vi "GetNoOfFilesandIndices.vi"(8 "error in (no error)":errorcluster, 10 "Partial Image File Name":string="cameraA-nr", 11 "File Path":path=path "Z:/Downloads/Fridge Pictures/1") -> (0 "error out":errorcluster, 1 "Number of Files":i32, 2 "max value":i32, 3 "min value":i32, 4 "Index number of Files":i32[](array[numeric]), 5 "Dt":u32)   [LabVIEW 2013]
doc: "Use this template to build a VI to use as a subVI."
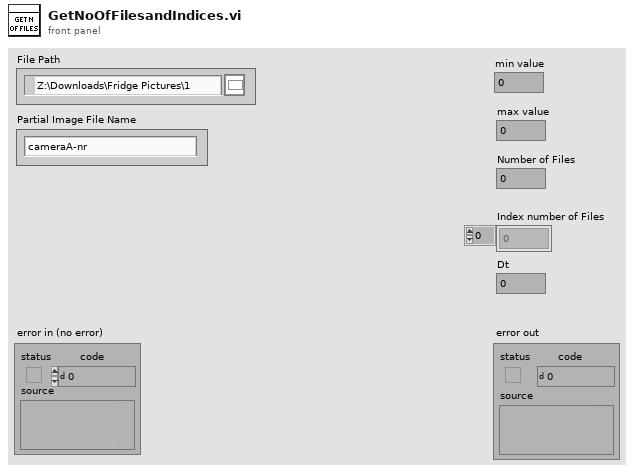
[diagram p1: front panel]
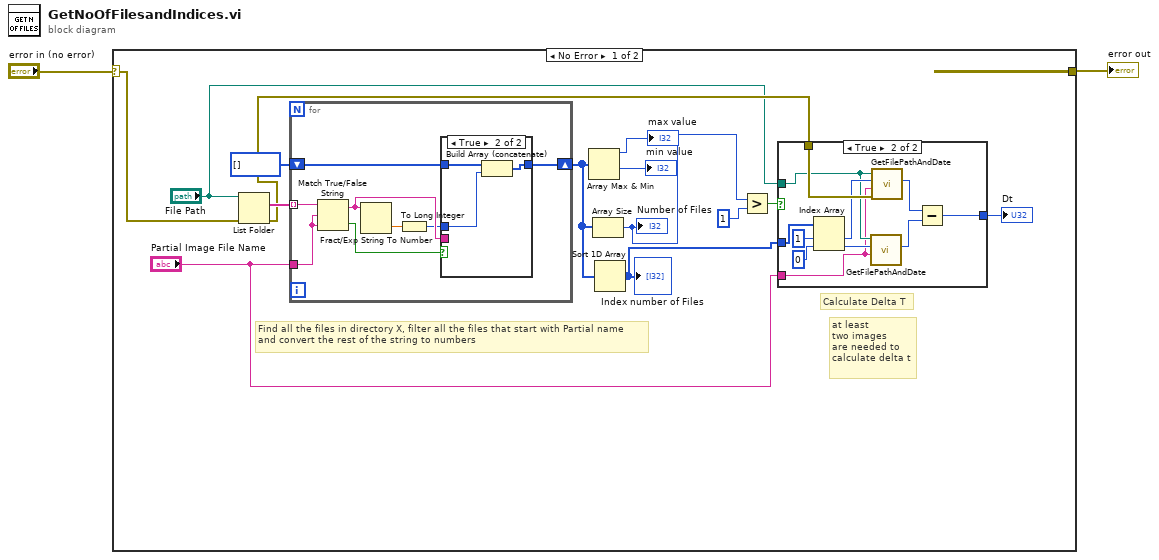
[diagram p0: block diagram]
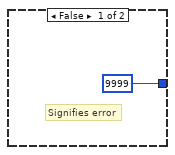
[diagram p2: hidden frame]
diagram:
  n1 = case shown="No Error" "error in (no error)" {
    selector: "error in (no error)" -> [w12 w41]
    tunnel: [_ w41] -> w1
    frame No Error {
      # "at least\ntwo images\nare needed to \ncalculate delta t"
      # "Calculate Delta T"
      # "Find all the files in directory X, filter all the files that start with Partial name\nand convert the rest of the string to numbers"
      n2 = List Folder(path="File Path", error in=w12) -> (filenames=w16:string[], error out=w10:errorcluster)  [unwired: 2 in, 2 out]
      n3 = for {
        tunnel: w16 -> [w36] mode=indexing
        tunnel: "Partial Image File Name" -> [w32]
        shift-right: [w35] -> w13
        shift-left: i32[] [] -> [w34]
        n4 = Match True/False String(2:w32, 3:w32, 4:w36) -> (0:w33:bool, 1:w31:string)
        n5 = Fract/Exp String To Number(string=w31) -> (number=w30:dbl)  [unwired: 3 in, 1 out]
        n6 = To Long Integer(number=w30) -> (32bit integer=w29:i32)
        n7 = case shown="True" w33 {
          tunnel: w31 -> [_ _]
          tunnel: [w37 w40] -> w35
          tunnel: w34 -> [w37 w39]
          tunnel: w29 -> [_ w38]
          frame False {
          }
          frame True {
            n8 = Build Array (concatenate)(w39, w38) -> (w40:i32[])
          }
        }
      }
      n9 = Array Max & Min(array=w13) -> (max value=→"max value":i32, min value=→"min value":i32)  [unwired: 2 out]
      n10 = Array Size(array=w13) -> (size(s)=w9:i32)
      "Number of Files" <- w9
      n11 = Sort 1D Array(array=w13) -> (sorted array=w6:i32[])
      "Index number of Files" <- w6
      n12 = Greater?(x=w9, y=1) -> (0:w7:bool)
      n13 = case shown="True" w7 {
        tunnel: w10 -> [_ w28]
        tunnel: w6 -> [_ w27]
        tunnel: "File Path" -> [_ w22]
        tunnel: "Partial Image File Name" -> [_ w21]
        tunnel: [u32 9999 w18] -> w3
        frame False {
          # "Signifies error"
        }
        frame True {
          n14 = Index Array(array=w27, index #1=1 ("index"), index #2=0 ("index")) -> (element #1=w24:i32, element #2=w23:i32)
          n15 = call "GetFilePathAndDate.vi"("String"=w21, "Index"=w23, "Path"=w22) -> ("creation date"=w19:u32)  [unwired: 6 in, 2 out]
          n16 = call "GetFilePathAndDate.vi"("error in (no error)"=w28, "String"=w21, "Index"=w24, "Path"=w22) -> ("creation date"=w20:u32)  [unwired: 5 in, 2 out]
          n17 = Subtract(x=w20, y=w19) -> (x-y=w18:u32)
        }
      }
      "Dt" <- w3
    }
    frame Error {
    }
  }
  "error out" <- w1
